vi "High Scores.vi"(10 "Reset?":bool, 11 "Player Data":T1) -> (3 "Table":string[][](table))   [LabVIEW 2014]
panel:
  out "element 2":i32
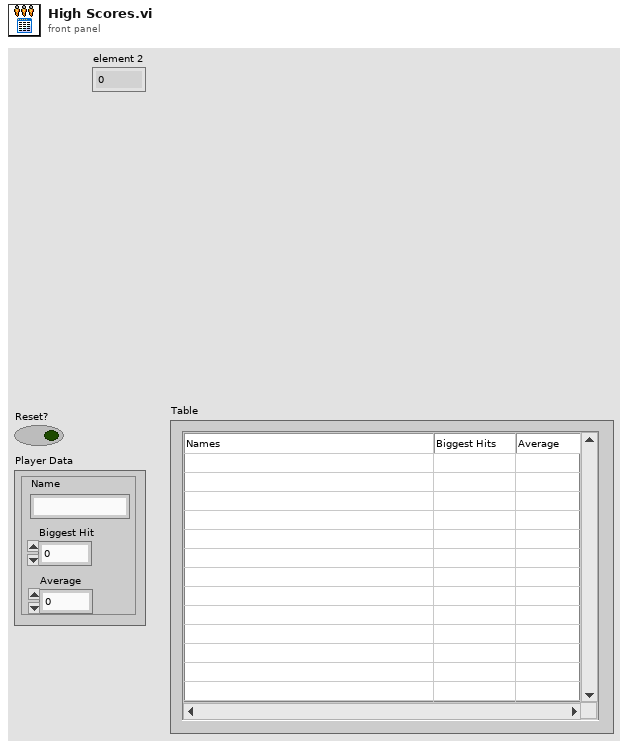
[diagram p1: front panel]
types:
  T1 = cluster{"Name":string, "Biggest Hit":dbl, "Average":dbl}
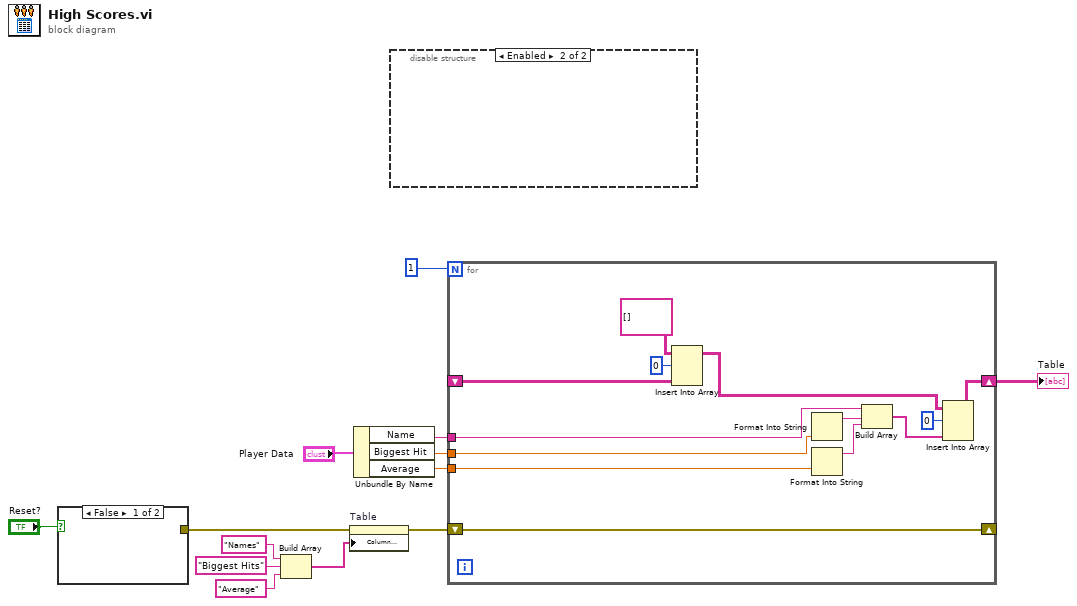
[diagram p0: block diagram]
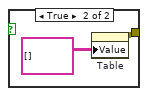
[diagram p2: hidden frame]
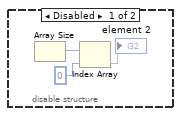
[diagram p3: hidden frame]
diagram:
  n1 = case shown="False" "Reset?" {
    tunnel: [_ w14] -> w3
    frame False {
    }
    frame True {
      n2 = property on="Table" class="Tbl (strict)"("Value"=string[][] [] ("array")) -> (error out=w14:errorcluster)  [unwired: 2 in, 1 out]
    }
  }
  n3 = Build Array("Names", "Biggest Hits" ("element"), "Average" ("element")) -> (w1:string[])
  n4 = property on="Table" class="Tbl (strict)"(error in=w3, "Column Headers[]"=w1) -> (error out=w2:errorcluster)  [unwired: 1 in, 1 out]
  n5 = Unbundle By Name("Player Data") -> ("Name"=w7:string, "Biggest Hit"=w6:dbl, "Average"=w5:dbl)
  n6 = disable-structure shown="Enabled" {
    frame Disabled {
      n7 = Array Size() -> (size(s)=w16:i32)  [unwired: 1 in]
      n8 = Index Array(array=w16, index=0) -> (element=→"element 2")
    }
    frame Enabled {
    }
  }
  n9 = for {
    N: 1 -> [_]
    tunnel: w7 -> [w31]
    tunnel: w6 -> [w30]
    tunnel: w5 -> [w28]
    shift-right: [w23] -> w13
    shift-left: _ -> [w25]
    shift-right: [w20] -> _
    shift-left: w2 -> [w20]
    n10 = Insert Into Array(array=string[][] [], index (row)=0, new element=w25) -> (w22:string[][])  [unwired: 1 in]
    n11 = Format Into String(w30) -> (resulting string=w29:string)  [unwired: 3 in, 1 out]
    n12 = Format Into String(w28) -> (resulting string=w27:string)  [unwired: 3 in, 1 out]
    n13 = Build Array(w31, w29, w27) -> (w26:string[])
    n14 = Insert Into Array(array=w22, index (row)=0, new element=w26) -> (w23:string[][])  [unwired: 1 in]
  }
  "Table" <- w13
